vi "counter_with_reset.vi"(1 "reset":bool) -> (0 "count":u32)   [LabVIEW 2018]
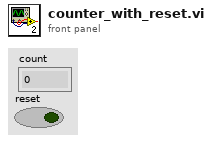
[diagram p1: front panel]
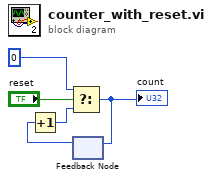
[diagram p0: block diagram]
diagram:
  n1 = feedback #1() -> (w3:u32)  [unwired: 1 in]
  n2 = Increment(x=w3) -> (x+1=w1:u32)
  n3 = Select(t=u32 0, s="reset", f=w1) -> (s? t:f=w2:u32)
  "count" <- w2
  n4 = feedback-in #1(w2) -> ()
